vi "Imaging DRAM Address Control.vi"(10 "output valid?":bool, 11 "Imaging DRAM address in":u32) -> (3 "Imaging DRAM address out":u32)   [LabVIEW 2015]
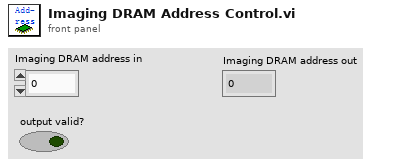
[diagram p1: front panel]
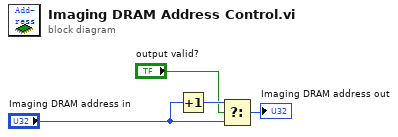
[diagram p0: block diagram]
diagram:
  n1 = Increment(x="Imaging DRAM address in") -> (x+1=w2:u32)
  n2 = Select(t=w2, s="output valid?", f="Imaging DRAM address in") -> (s? t:f=→"Imaging DRAM address out":u32)
